vi "RSZVB Get Calibration Type.vi"(0 "VISA session":refnum<visa-resource-name>, 5 "Channel (1)":i32=1, 11 "error in (no error)":errorcluster {"code" format="%.0x"}) -> (3 "Calibration Type":i32, 4 "dup VISA session":refnum<visa-resource-name>, 6 "Port 1":i32, 8 "Port 2":i32, 10 "Port 3":i32, 14 "Port 4":i32, 15 "error out":errorcluster {"code" format="%.0x"})   [LabVIEW 2011]
doc: "This VI returns the current calibration type. Returns the calibration type and the port numbers valid for that calibration.\n\nRemote-control command(s):\n[SENSe<Ch>:]CORRection:COLLect:METHod:DEFine?"
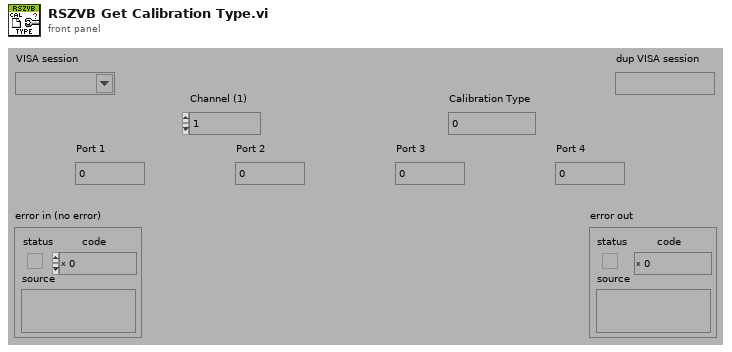
[diagram p1: front panel]
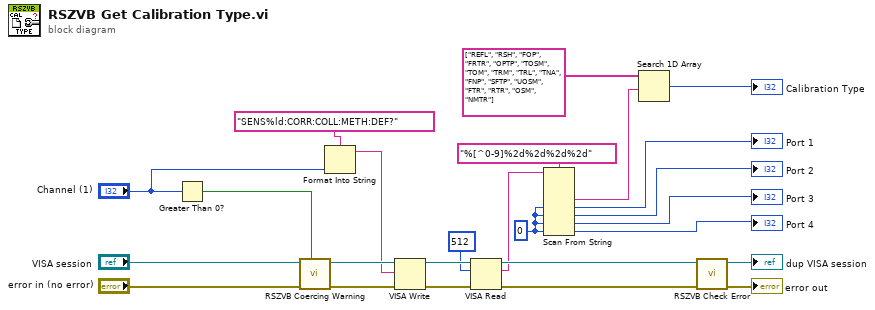
[diagram p0: block diagram]
diagram:
  w8 = 0 ("default value 5")
  n1 = Greater Than 0?(x="Channel (1)") -> (x > 0?=w17:bool)
  n2 = call "RSZVB Coercing Warning.vi"("In Range?"=w17, "error in (no error)"="error in (no error)", "VISA session"="VISA session") -> ("error out"=w24:errorcluster, "dup VISA session"=w25:refnum<visa-resource-name>)  [unwired: 7 in]
  n3 = Format Into String(format string="SENS%ld:CORR:COLL:METH:DEF?", "Channel (1)") -> (resulting string=w12:string)  [unwired: 2 in, 1 out]
  n4 = VISA Write(VISA resource name=w25, write buffer=w12, error in (no error)=w24) -> (VISA resource name out=w23:refnum<visa-resource-name>, error out=w22:errorcluster)  [unwired: 1 out]
  n5 = VISA Read(VISA resource name=w23, byte count=u32 512 ("byte count (0)"), error in (no error)=w22) -> (VISA resource name out=w21:refnum<visa-resource-name>, read buffer=w10:string, error out=w20:errorcluster)  [unwired: 1 out]
  n6 = Scan From String(format string="%[^0-9]%2d%2d%2d%2d", input string=w10, default 2=w8, default 3=w8, default 4=w8, default 5=w8) -> (output 1=w6:string, output 2=→"Port 1":i32, output 3=→"Port 2":i32, output 4=→"Port 3":i32, output 5=→"Port 4":i32)  [unwired: 3 in, 3 out]
  n7 = Search 1D Array(1D array=string[] ["REFL", "RSH", "FOP", "FRTR", "OPTP", "TOSM", "TOM", "TRM", "TRL", "TNA", "FNP", "SFTP", "UOSM", "FTR", "RTR", "OSM", "NMTR"] ("array"), element=w6) -> (index of element=→"Calibration Type":i32)  [unwired: 1 in]
  n8 = call "RSZVB Check Error.vi"("error in (no error)"=w20, "VISA session"=w21) -> ("error out"=→"error out":errorcluster, "dup VISA session"=→"dup VISA session":refnum<visa-resource-name>)  [unwired: 8 in]
